vi "MDI_global.vi"() -> ()   [LabVIEW 2009]
panel:
  out "VI Ref container":refnum<vi>
  out "container_Wnd":u32
  out "main_wnd":u32
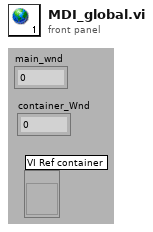
[diagram p1: front panel]
diagram:
